vi "Get Image.vi"() -> ()   [LabVIEW 2013]
uses:
  <vilib>/vision/driver/NI_Vision_Acquisition_Software.lvlib
  <vilib>/vision/NI_Vision_Development_Module.lvlib
  <vilib>/userdefined/High Color/IMAQdx.ctl
panel:
  out "Real Image":T1(plugin-control)
  out "Raw Image":T1(plugin-control)
  in  "stop":bool
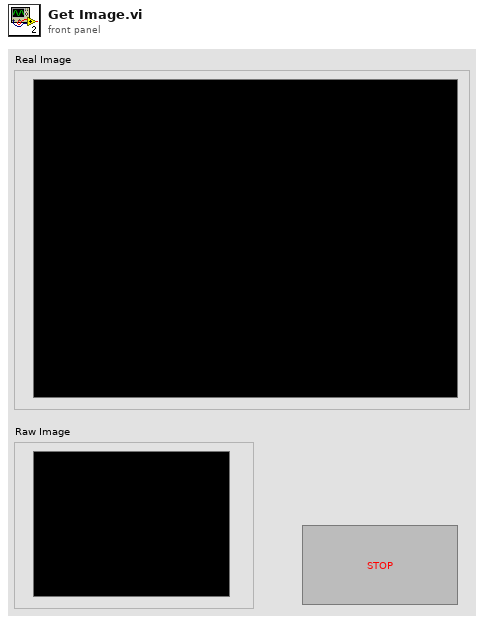
[diagram p1: front panel]
types:
  T1 = typedef "IMAQ Image.ctl" = refnum<image>
  T2 = typedef "IMAQdx.ctl" = refnum<k21>
  T3 = cluster{"Position":cluster{"x":sgl, "y":sgl}, "Angle":sgl, "Scale":sgl, "Score":sgl, "Bounding Box":cluster{"x":sgl, "y":sgl}[]}[]
  T4 = cluster{"Position":cluster{"x":sgl, "y":sgl}, "Angle":sgl, "Scale":sgl, "Score":sgl, "Bounding Box":cluster{"x":sgl, "y":sgl}[]}
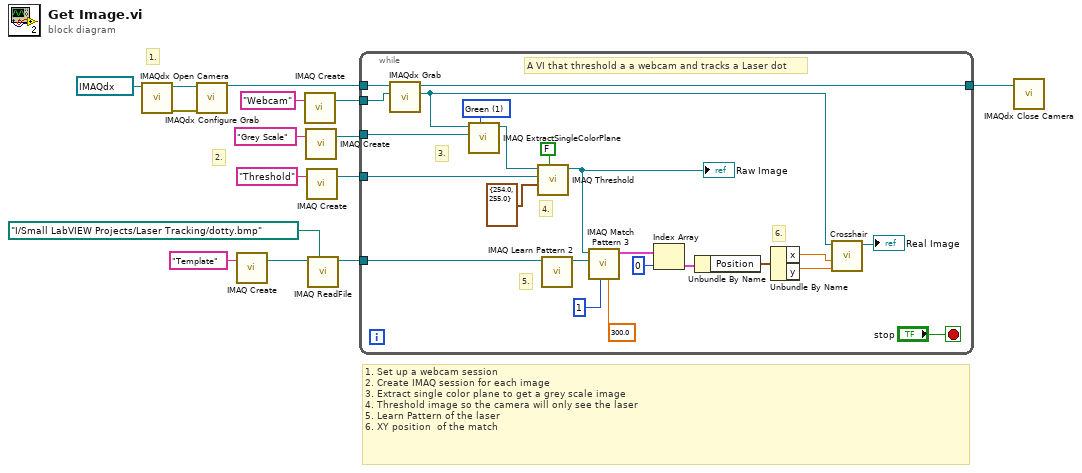
[diagram p0: block diagram]
diagram:
  # "1. Set up a webcam session\n2. Create IMAQ session for each image\n3. Extract single color plane to get a grey scale image\n4. Threshold image so the camera will only see the laser\n5. Learn Pattern of the laser\n6. XY position  of the match"
  # "2."
  # "1."
  n1 = call <vilib>:"IMAQdx Open Camera.vi"("Session In"=T2 "cam0") -> ("error out"=w1:errorcluster, "Session Out"=w15:T2)  [unwired: 9 in]
  n2 = call <vilib>:"IMAQdx Configure Grab.vi"("error in"=w1, "Session In"=w15) -> ("Session Out"=w8:T2)  [unwired: 8 in, 1 out]
  n3 = call "IMAQ Create"("Image Name"="Template") -> ("New Image"=w10:T1)  [unwired: 4 in, 1 out]
  n4 = call "IMAQ Create"("Image Name"="Webcam") -> ("New Image"=w6:T1)  [unwired: 4 in, 1 out]
  n5 = call "IMAQ Create"("Image Name"="Grey Scale") -> ("New Image"=w5:T1)  [unwired: 4 in, 1 out]
  n6 = call "IMAQ Create"("Image Name"="Threshold") -> ("New Image"=w4:T1)  [unwired: 4 in, 1 out]
  n7 = call "IMAQ ReadFile"("File Path"=path "I:/Small LabVIEW Projects/Laser Tracking/dotty.bmp", "Image"=w10) -> ("Image Out"=w3:T1)  [unwired: 5 in, 4 out]
  n8 = while {
    tunnel: w8 -> [w38]
    tunnel: w6 -> [w37]
    tunnel: [w36] -> w2
    tunnel: w5 -> [w35]
    tunnel: w4 -> [w32]
    tunnel: w3 -> [w20]
    stop <- "stop" stop-if-true
    w34 = 1 items=["Red", "Green", "Blue", "Hue", "Saturation", "Luminance", "Value", "Intensity"] ("Color Plane")
    # "6."
    # "5."
    # "4."
    # "3."
    # "A VI that threshold a a webcam and tracks a Laser dot"
    n9 = call <vilib>:"IMAQdx Grab.vi"("Image In"=w37, "Session In"=w38) -> ("Image Out"=w17:T1, "Session Out"=w36:T2)  [unwired: 6 in, 2 out]
    n10 = call "IMAQ ExtractSingleColorPlane"("Color Plane"=w34, "Image Dst"=w35, "Image Src"=w17) -> ("Image Dst Out"=w33:T1)  [unwired: 7 in, 1 out]
    n11 = call "IMAQ Threshold"("Keep/Replace Value (Replace)"=FALSE, "Range"=cluster{"Lower value":sgl, "Upper value":sgl} {"Lower value"=254.0, "Upper value"=255.0}, "Image Dst"=w32, "Image Src"=w33) -> ("Image Dst Out"=w21:T1)  [unwired: 6 in, 1 out]
    "Raw Image" <- w21
    n12 = call "IMAQ Learn Pattern 2"("Image"=w20) -> ("Template Image Out"=w29:T1)  [unwired: 9 in, 1 out]
    n13 = call "IMAQ Match Pattern 3"("Minimum Match Score"=sgl 300.0, "Number of Matches Requested"=1, "Template Image"=w29, "Image"=w21) -> ("Matches"=w26:T3)  [unwired: 5 in, 2 out]
    n14 = Index Array(array=w26, index=0) -> (element=w24:T4)
    n15 = Unbundle By Name(w24) -> ("Position"=w22:cluster{"x":sgl, "y":sgl})
    n16 = Unbundle By Name(w22) -> ("x"=w19:sgl, "y"=w18:sgl)
    n17 = call "Crosshair.vi"("Y"=w18, "X"=w19, "Webcam In"=w17) -> ("Webcam out"=→"Real Image":T1)  [unwired: 8 in]
  }
  n18 = call <vilib>:"IMAQdx Close Camera.vi"("Session In"=w2) -> ()  [unwired: 10 in, 1 out]
